vi "ConvertLUTToLVLUT.vi"(9 "LUT":sgl[][](array[numeric]), 10 "width":u32, 11 "minRadius":sgl) -> (3 "LV tracker rad prof":dbl[][](array[numeric]))   [LabVIEW 2011]
uses:
  qtrk/QTrkLVBinding/XYZf.ctl
panel:
  out "Radial Profile":dbl[](graph)
  out "Image":sgl[][](graph)
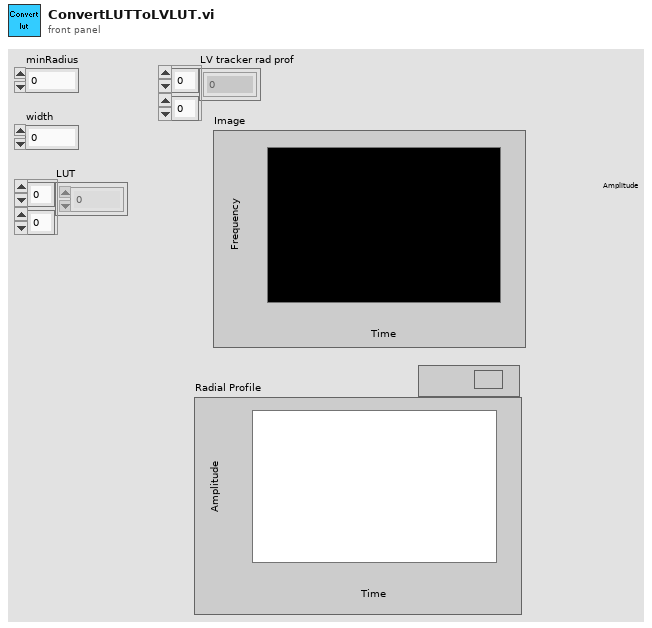
[diagram p1: front panel]
types:
  T1 = cluster{"Rmax (pix)":i32, "RminZ (pix)":i32, "angular pixel\n coverage factor":dbl, "radial pixel\n coverage factor":dbl}
  T2 = typedef "XYZf.ctl" = cluster{"X":sgl, "Y":sgl, "Z":sgl}
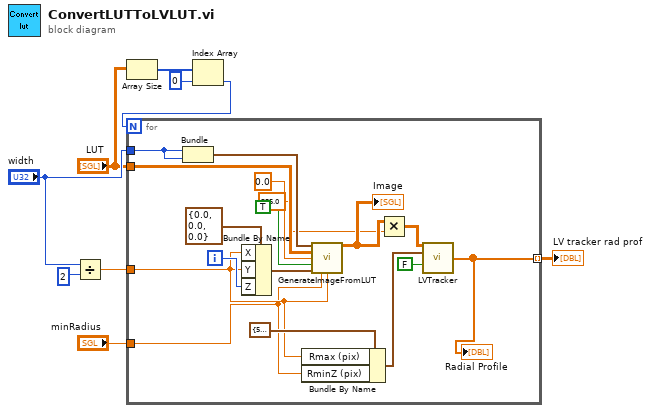
[diagram p0: block diagram]
diagram:
  n1 = Divide(x="width", y=u32 2) -> (x/y=w6:dbl)
  n2 = Array Size(array="LUT") -> (size(s)=w2:i32[])
  n3 = Index Array(array=w2, index=0) -> (element=w1:i32)
  n4 = for {
    N: w1 -> [_]
    tunnel: "LUT" -> [w26]
    tunnel: "width" -> [w22]
    tunnel: w6 -> [w16]
    tunnel: "minRadius" -> [w15]
    tunnel: [w13] -> w9 mode=indexing
    i -> [w24]
    n5 = Bundle("width"=w22, "width"=w22) -> (w23:cluster{"width":u32, "width":u32})  [unwired: 1 in]
    n6 = Bundle By Name(cluster=T2 {"X"=0.0, "Y"=0.0, "Z"=0.0} ("XYZ"), "X"=w16, "Y"=w16, "Z"=w24) -> (w20:T2)
    n7 = Bundle By Name(cluster=T1 {"Rmax (pix)"=50, "RminZ (pix)"=5, "angular pixel\n coverage factor"=0.7, "radial pixel\n coverage factor"=3.0} ("settings"), "Rmax (pix)"=w16, "RminZ (pix)"=w15) -> (w17:T1)
    n8 = call "GenerateImageFromLUT.vi"("Image Size"=w23, "ZLUT"=w26, "Pixel max value"=sgl 0.0, "Use spline interpolation?"=TRUE, "XYZ"=w20, "ZLUT MinRadius"=w15, "ZLUT MaxRadius"=w16) -> ("Result image"=w12:sgl[][])  [unwired: 8 in]
    "Image" <- w12
    n9 = Multiply(x=w12, y=sgl 255.0 ("Pixel max value")) -> (x*y=w10:sgl[][])
    n10 = call "LVTracker.vi"("image in"=w10, "settings"=w17, "Compute Z"=FALSE) -> ("LV tracker rad prof"=w13:dbl[])  [unwired: 5 in, 7 out]
    "Radial Profile" <- w13
  }
  "LV tracker rad prof" <- w9
